vi "HW XML Tx - Write.vi"(0 "String (in)":string, 1 "Use Octal Channel Names?":bool, 2 "Selected Channels":i32[](array[numeric]), 5 "formatting (NIVeriStandAdd-Ons)":enum16{"NIVeriStandAdd-Ons", "ni"}(ring), 7 "Parameter Array":T1[](array[typedef])) -> (4 "String (out)":string)   [LabVIEW 2020]
uses:
  Controls/Database_Array.ctl
  Controls/Encoding.ctl
  <userlib>/_OpenG.lib/array/array.llb/Remove Duplicates from 1D Array (I32)__ogtk.vi
  <userlib>/_OpenG.lib/array/array.llb/Filter 1D Array with Scalar (I32)__ogtk.vi
  <userlib>/_OpenG.lib/array/array.llb/Index 1D Array Elements (Variant)__ogtk.vi
  <userlib>/_OpenG.lib/array/array.llb/Remove Duplicates from 1D Array (U32)__ogtk.vi
  <userlib>/_OpenG.lib/array/array.llb/Filter 1D Array with Scalar (U32)__ogtk.vi
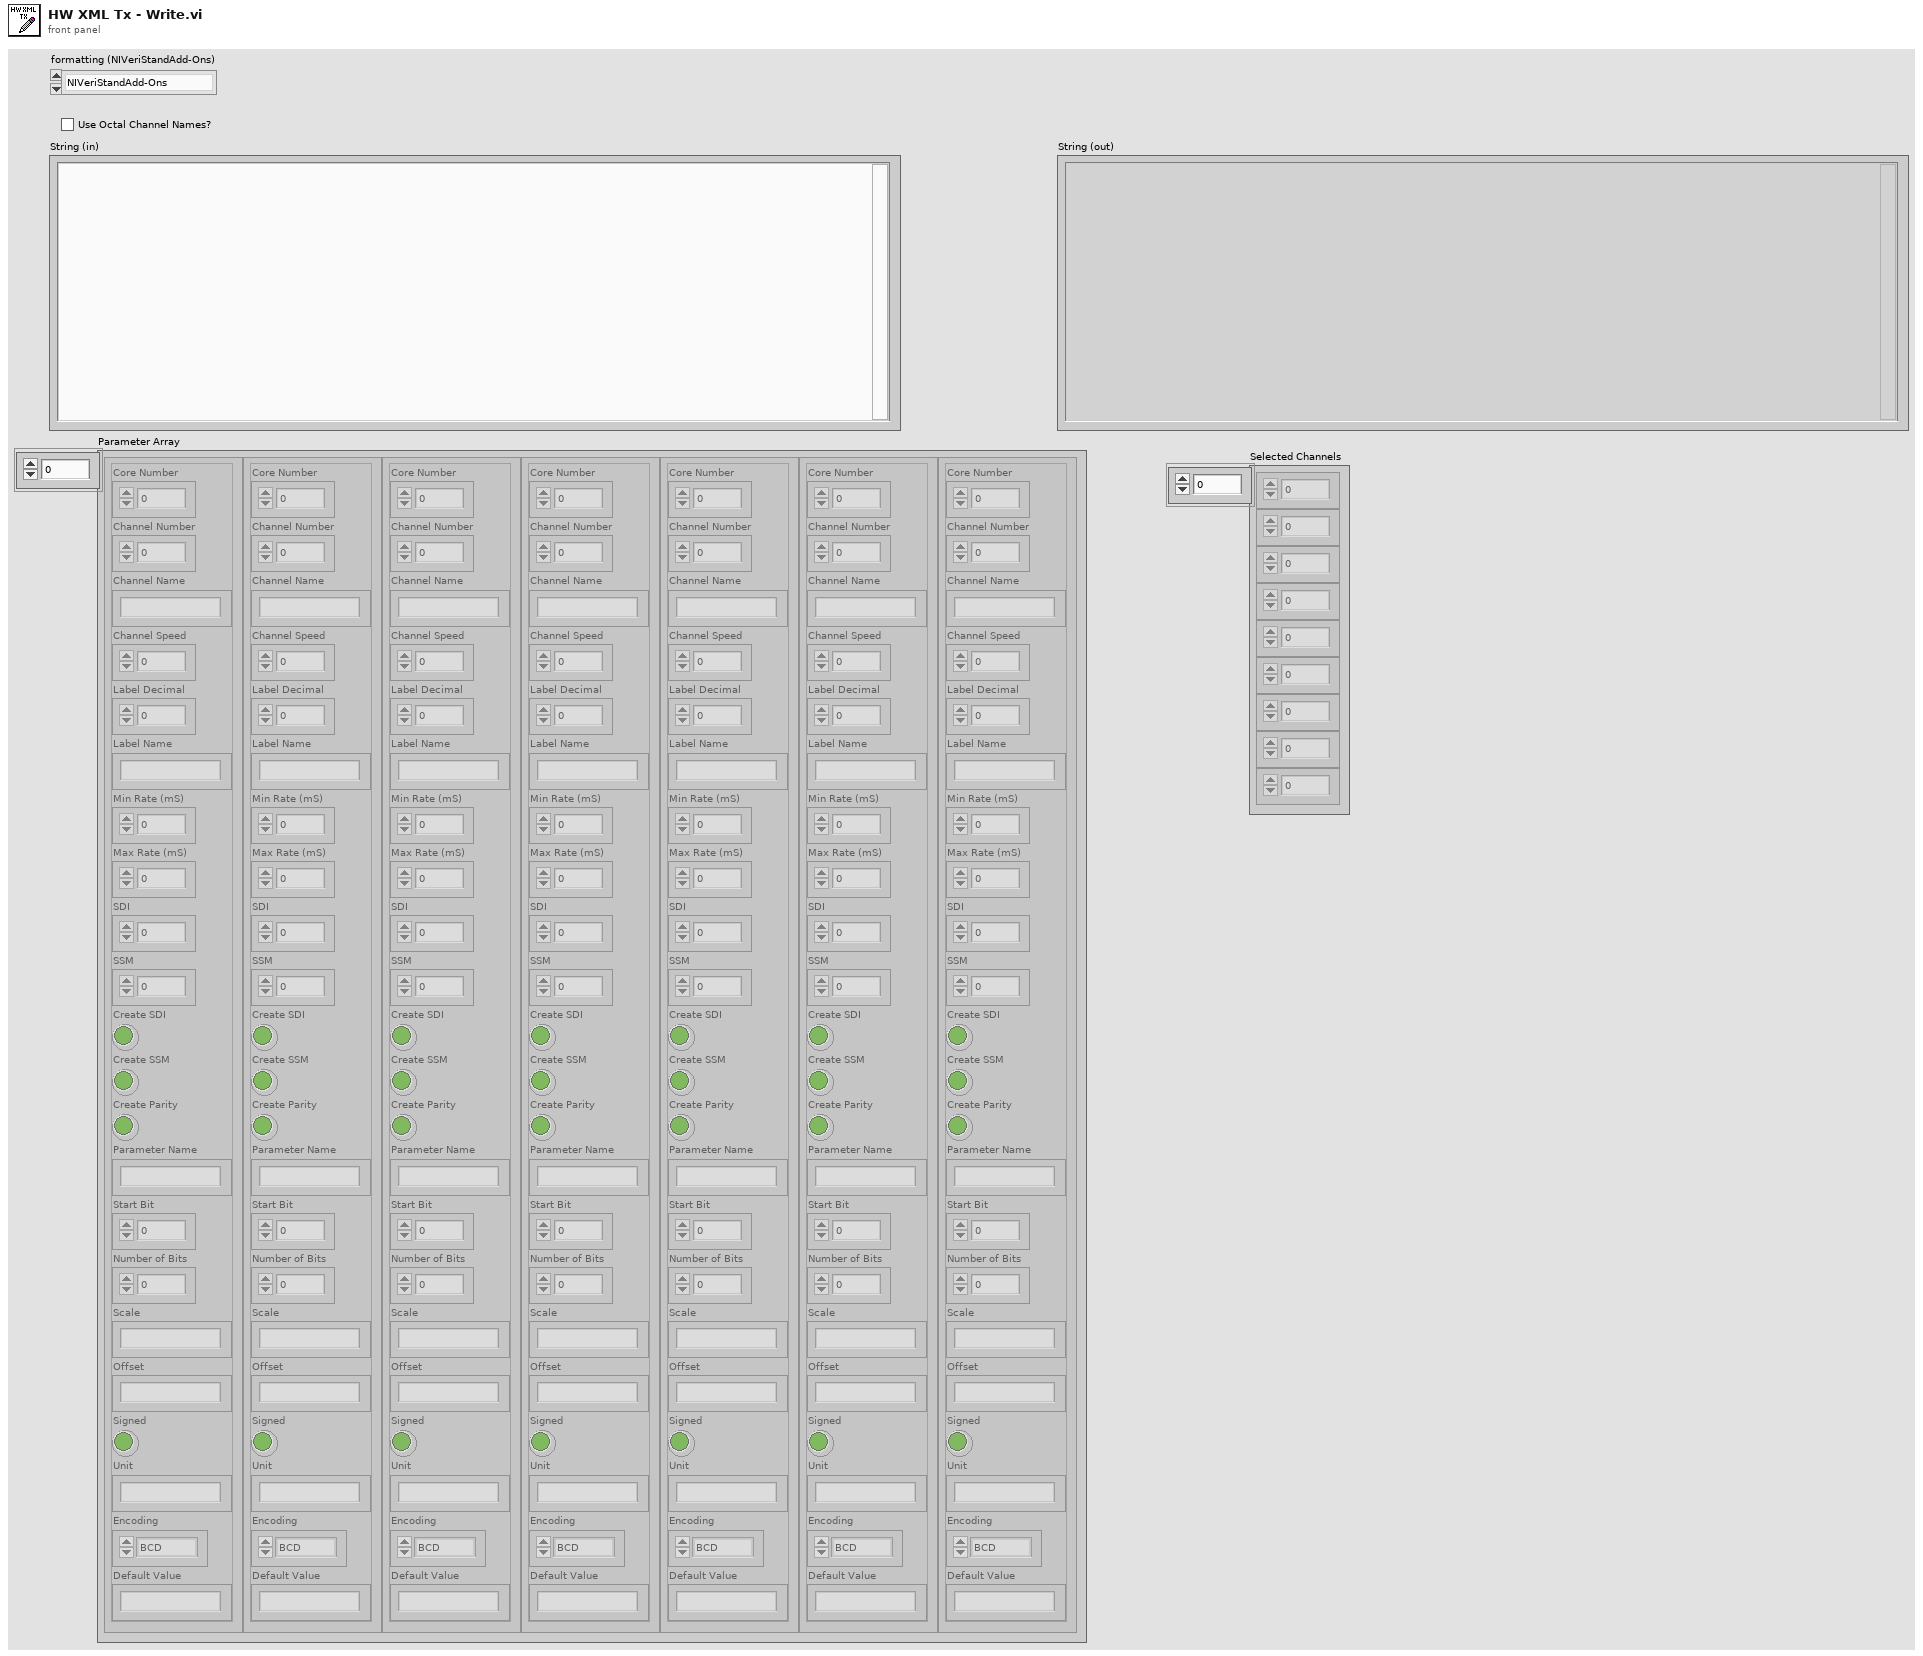
[diagram p1: front panel]
types:
  T1 = typedef "Database_Array.ctl" = cluster{"Core Number":i32, "Channel Number":i32, "Channel Name":string, "Channel Speed":i32, "Label Decimal":u32, "Label Name":string, "Min Rate (mS)":i32, "Max Rate (mS)":i32, "SDI":i32, "SSM":i32, "Create SDI":bool, "Create SSM":bool, "Create Parity":bool, "Parameter Name":string, "Start Bit":i32, "Number of Bits":i32, "Scale":string, "Offset":string, "Signed":bool, "Unit":string, "Encoding":T2, "Default Value":string}
  T2 = typedef "Encoding.ctl" = enum16{"BCD", "BNR", "Discrete"}
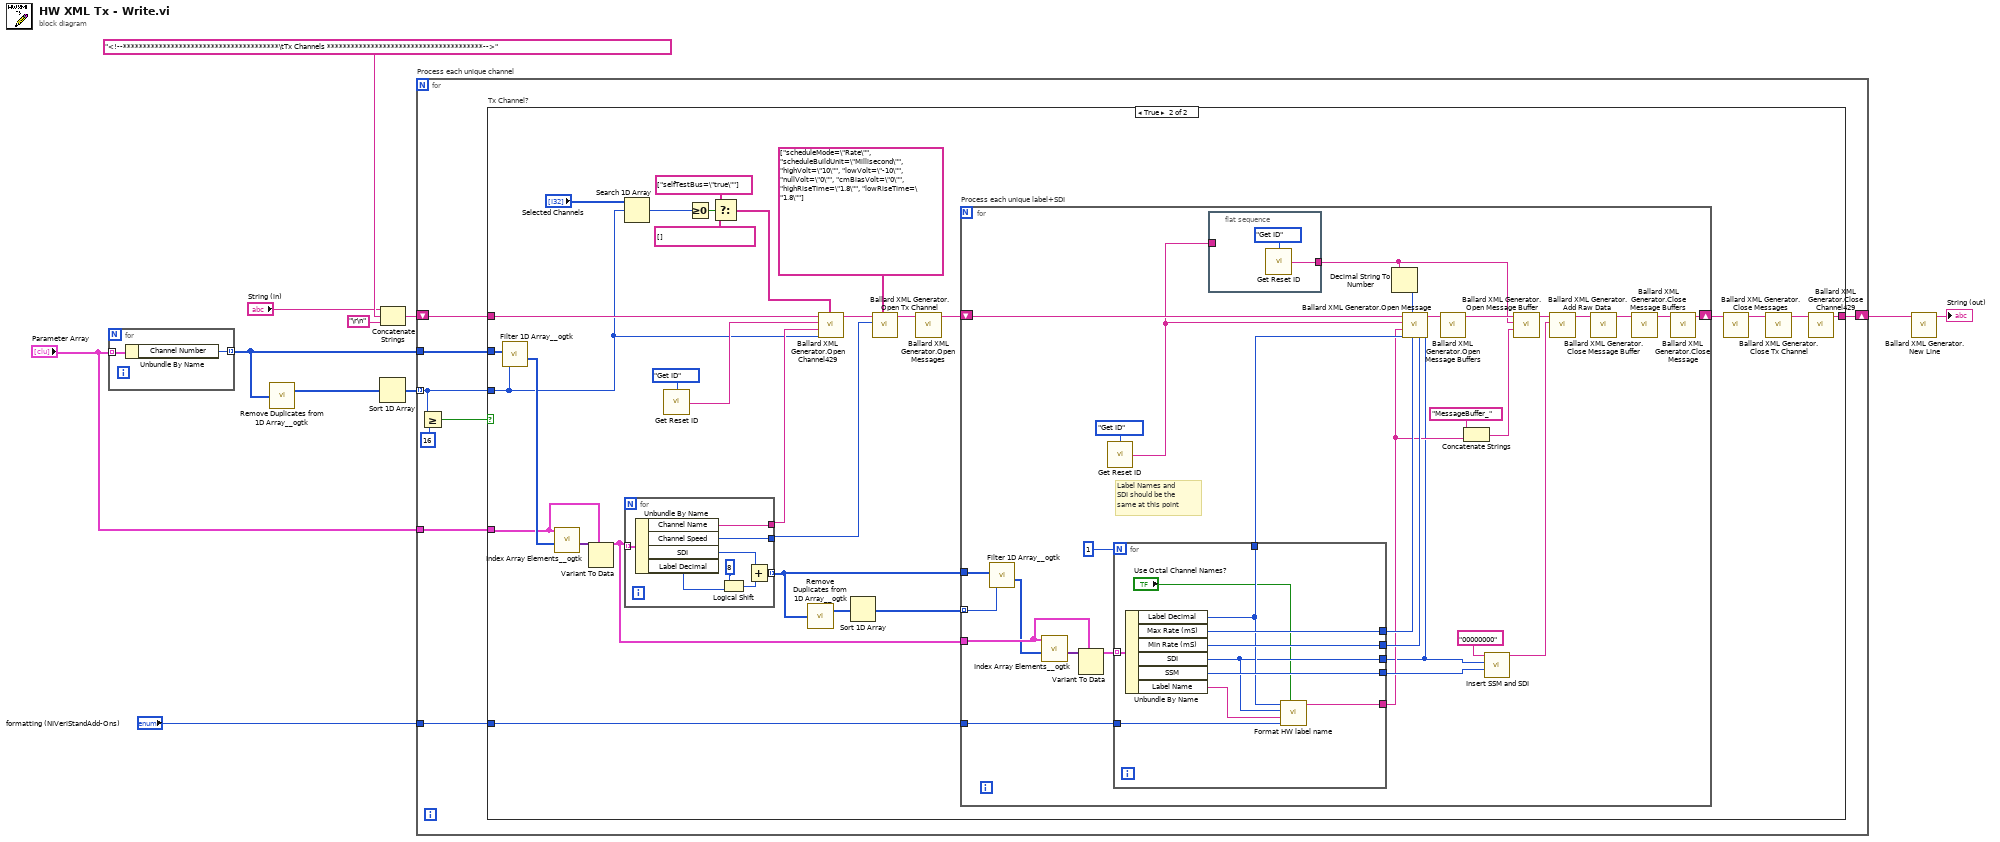
[diagram p0: block diagram]
diagram:
  n1 = for {
    tunnel: [w13] -> w3 mode=indexing
    tunnel: "Parameter Array" -> [w12] mode=indexing
    n2 = Unbundle By Name(w12) -> ("Channel Number"=w13:i32)
  }
  n3 = call-poly <userlib>:"Remove Duplicates from 1D Array__ogtk.vi"("Input Array"=w3) -> ("Output Array"=w10:i32[])  [unwired: 1 out]
  n4 = Sort 1D Array(array=w10) -> (sorted array=w11:i32[])
  n5 = Concatenate Strings("String (in)", "<!--***************************************\tTx Channels ***************************************-->", "\r\n") -> (w7:string)
  n6 = for "Process each unique channel" {
    tunnel: w11 -> [w18] mode=indexing
    tunnel: w3 -> [w21]
    shift-right: [w19] -> w2
    shift-left: w7 -> [w20]
    tunnel: "Parameter Array" -> [w15]
    tunnel: "formatting (NIVeriStandAdd-Ons)" -> [w14]
    n7 = Greater Or Equal?(x=w18, y=16) -> (x >= y?=w17:bool)
    n8 = case "Tx Channel?" shown="True" w17 {
      tunnel: w21 -> [_ w51]
      tunnel: w20 -> [w22 w48]
      tunnel: [w22 w41] -> w19
      tunnel: w18 -> [_ w25]
      tunnel: w15 -> [_ w35]
      tunnel: w14 -> [_ w23]
      frame False {
      }
      frame True {
        n9 = call-poly <userlib>:"Filter 1D Array__ogtk.vi"("items to filter"=w25, "array"=w51) -> ("filtered item indices"=w39:i32[])  [unwired: 4 in, 1 out]
        n10 = call-poly <userlib>:"Index Array Elements__ogtk.vi"("indices"=w39, "array"=w35) -> ("elements"=w38:variant[])  [unwired: 9 in]
        n11 = Variant To Data(type=w35, Variant=w38) -> (data=w34:T1[])  [unwired: 1 in, 1 out]
        n12 = Search 1D Array(1D array="Selected Channels", element=w25) -> (index of element=w29:i32)  [unwired: 1 in]
        n13 = for {
          tunnel: w34 -> [w59] mode=indexing
          tunnel: [w58] -> w37
          tunnel: [w57] -> w36
          tunnel: [w52] -> w33 mode=indexing
          n14 = Unbundle By Name(w59) -> ("Channel Name"=w58:string, "Channel Speed"=w57:i32, "SDI"=w54:i32, "Label Decimal"=w53:u32)
          n15 = Logical Shift(y=i16 8, x=w53) -> (x << y=w56:u32)
          n16 = Add(x=w54, y=w56) -> (x+y=w52:u32)
        }
        n17 = call "Get Reset ID.vi"("Function"=enum16{"Get ID", "Reset ID"}."Get ID") -> ("ID"=w32:string)  [unwired: 14 in]
        n18 = Greater Or Equal To 0?(x=w29) -> (x >= 0?=w30:bool)
        n19 = Select(t=string[] ["selfTestBus=\"true\""] ("other params"), s=w30, f=string[] [] ("other params")) -> (s? t:f=w24:string[])
        n20 = call-poly <userlib>:"Remove Duplicates from 1D Array__ogtk.vi"("Input Array"=w33) -> ("Output Array"=w50:u32[])  [unwired: 1 out]
        n21 = call "Ballard XML Generator.Open Channel429.vi"("other params"=w24, "hardware channel"=w25, "name"=w37, "id"=w32, "string in"=w48) -> ("string out"=w46:string)  [unwired: 6 in]
        n22 = Sort 1D Array(array=w50) -> (sorted array=w49:u32[])
        n23 = call "Ballard XML Generator.Open Tx Channel.vi"("other params"=string[] ["scheduleMode=\"Rate\"", "scheduleBuildUnit=\"Millisecond\"", "highVolt=\"10\"", "lowVolt=\"-10\"", "nullVolt=\"0\"", "cmBiasVolt=\"0\"", "highRiseTime=\"1.8\"", "lowRiseTime=\"1.8\""], "speedKHz"=w36, "string in"=w46) -> ("string out"=w47:string)  [unwired: 8 in]
        n24 = call "Ballard XML Generator.Open Messages.vi"("string in"=w47) -> ("string out"=w45:string)  [unwired: 10 in]
        n25 = for "Process each unique label+SDI" {
          tunnel: w49 -> [w87] mode=indexing
          tunnel: w33 -> [w89]
          shift-right: [w78] -> w44
          shift-left: w45 -> [w88]
          tunnel: w34 -> [w71]
          tunnel: w23 -> [w60]
          # "Label Names and SDI should be the same at this point"
          n26 = call-poly <userlib>:"Filter 1D Array__ogtk.vi"("items to filter"=w87, "array"=w89) -> ("filtered item indices"=w70:i32[])  [unwired: 4 in, 1 out]
          n27 = call-poly <userlib>:"Index Array Elements__ogtk.vi"("indices"=w70, "array"=w71) -> ("elements"=w74:variant[])  [unwired: 9 in]
          n28 = Variant To Data(type=w71, Variant=w74) -> (data=w73:T1[])  [unwired: 1 in, 1 out]
          n29 = call "Get Reset ID.vi"("Function"=enum16{"Get ID", "Reset ID"}."Get ID") -> ("ID"=w61:string)  [unwired: 14 in]
          n30 = for {
            N: 1 -> [_]
            tunnel: w73 -> [w101] mode=indexing
            tunnel: [w100] -> w69
            tunnel: [w99] -> w68
            tunnel: [w96] -> w64
            tunnel: [w98] -> w67
            tunnel: [w97] -> w66
            tunnel: [w94] -> w65
            tunnel: w60 -> [w93]
            n31 = Unbundle By Name(w101) -> ("Label Decimal"=w97:u32, "Max Rate (mS)"=w100:i32, "Min Rate (mS)"=w99:i32, "SDI"=w96:i32, "SSM"=w98:i32, "Label Name"=w95:string)
            n32 = call "Format HW label name.vi"("Use Octal Channel Names?"="Use Octal Channel Names?", "formatting"=w93, "Label Name in"=w95, "SDI"=w96, "Label Decimal"=w97) -> ("Label Name out"=w94:string)  [unwired: 6 in]
          }
          n33 = flat-sequence {
            tunnel: [w91] -> w62
            tunnel: w61 -> [_]
            frame #0 {
              n34 = call "Get Reset ID.vi"("Function"=enum16{"Get ID", "Reset ID"}."Get ID") -> ("ID"=w91:string)  [unwired: 14 in]
            }
          }
          n35 = Decimal String To Number(string=w62) -> (number=w77:i32)  [unwired: 2 in, 1 out]
          n36 = call "Ballard XML Generator.Open Message.vi"("SDI"=w64, "minRate (400)"=w68, "maxRate (400)"=w69, "messageBufferIDRef (128)"=w77, "labelDecimal"=w66, "name"=w65, "id"=w61, "string in"=w88) -> ("string out"=w86:string)  [unwired: 3 in]
          n37 = call "Ballard XML Generator.Open Message Buffers.vi"("string in"=w86) -> ("string out"=w85:string)  [unwired: 10 in]
          n38 = Concatenate Strings("MessageBuffer_" ("name"), w65) -> (w83:string)
          n39 = call "Insert SSM and SDI.vi"("SSM"=w67, "SDI"=w64, "Hex (in)"="00000000" ("raw data")) -> ("Hex (out)"=w75:string)  [unwired: 8 in]
          n40 = call "Ballard XML Generator.Open Message Buffer.vi"("name"=w83, "id"=w62, "string in"=w85) -> ("string out"=w79:string)  [unwired: 8 in]
          n41 = call "Ballard XML Generator.Add Raw Data.vi"("raw data"=w75, "string in"=w79) -> ("string out"=w80:string)  [unwired: 9 in]
          n42 = call "Ballard XML Generator.Close Message Buffer.vi"("string in"=w80) -> ("string out"=w81:string)  [unwired: 10 in]
          n43 = call "Ballard XML Generator.Close Message Buffers.vi"("string in"=w81) -> ("string out"=w82:string)  [unwired: 10 in]
          n44 = call "Ballard XML Generator.Close Message.vi"("string in"=w82) -> ("string out"=w78:string)  [unwired: 10 in]
        }
        n45 = call "Ballard XML Generator.Close Messages.vi"("string in"=w44) -> ("string out"=w43:string)  [unwired: 10 in]
        n46 = call "Ballard XML Generator.Close Tx Channel.vi"("string in"=w43) -> ("string out"=w42:string)  [unwired: 10 in]
        n47 = call "Ballard XML Generator.Close Channel429.vi"("string in"=w42) -> ("string out"=w41:string)  [unwired: 10 in]
      }
    }
  }
  n48 = call "Ballard XML Generator.New Line.vi"("string in"=w2) -> ("string out"=→"String (out)":string)  [unwired: 10 in]
